vi "Timeout Phase.vi"(8 "error in (no error)":errorcluster, 11 "Programming Logic in":refnum<class "Programming Logic.lvclass">) -> (0 "error out":errorcluster, 3 "Programming Logic out":refnum<class "Programming Logic.lvclass">, 9 "Timer":u16, 10 "Temperature":u16)   [LabVIEW 2014, in "Files Library.lvlib" / "Programming Logic.lvclass"]
uses:
  Programming Logic.lvclass
  Programming Logic.lvclass/Programming Logic.ctl
  Files Library.lvlib
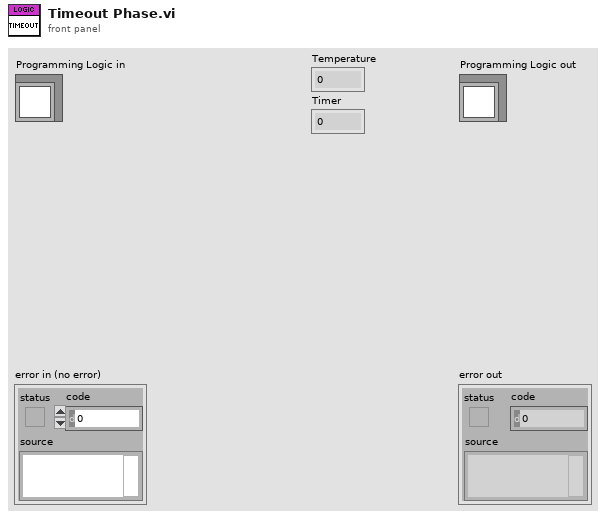
[diagram p1: front panel]
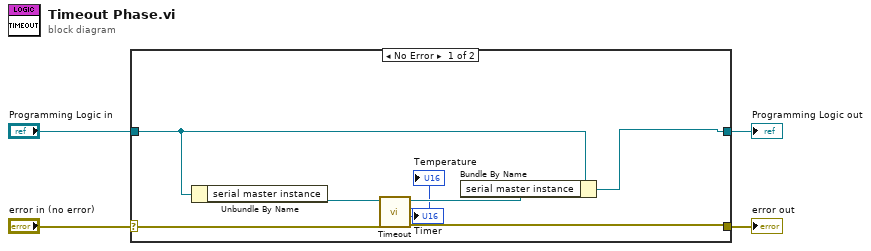
[diagram p0: block diagram]
diagram:
  n1 = case shown="No Error" "error in (no error)" {
    selector: "error in (no error)" -> [w8 w14]
    tunnel: [w7 w14] -> w3
    tunnel: [w9 w13] -> w1
    tunnel: "Programming Logic in" -> [w10 w13]
    frame No Error {
      n2 = Unbundle By Name(w10) -> ("serial master instance"=w12:refnum<class "Modbus Master.lvclass">)
      n3 = call "Timeout.vi"("error in"=w8, "Modbus master in"=w12) -> ("error out"=w7:errorcluster, "Modbus master out"=w11:refnum<class "Modbus Master.lvclass">, "Timer"=→"Timer":u16, "Temperature"=→"Temperature":u16)  [unwired: 6 in]
      n4 = Bundle By Name(cluster=w10, "serial master instance"=w11) -> (w9:refnum<class "Programming Logic.lvclass">)
    }
    frame Error {
    }
  }
  "error out" <- w3
  "Programming Logic out" <- w1
